vi "Start Synched Loops.vi"(8 "Error In":errorcluster) -> (0 "Error Out":errorcluster)   [LabVIEW 2014]
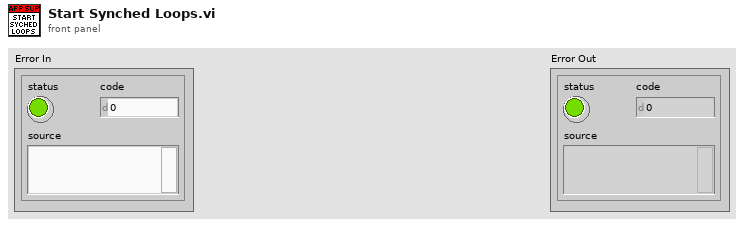
[diagram p1: front panel]
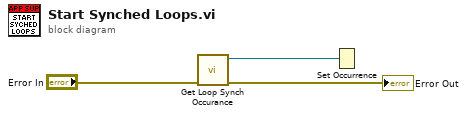
[diagram p0: block diagram]
diagram:
  n1 = call "Get Loop Synch Occurance.vi"("Error In"="Error In") -> ("Error Out"=→"Error Out":errorcluster, "Loop Synch Occourance"=w1:refnum<k4>)  [unwired: 9 in]
  n2 = Set Occurrence(w1) -> ()
